vi "MH_WRabbitSetSFPData.vi"(6 "alphas":i32[](array[numeric]), 7 "sfpnames":string[](array[string]), 8 "error in (no error)":errorcluster, 9 "dRxs":i32[](array[numeric]), 10 "dTxs":i32[](array[numeric]), 11 "devidx":i32) -> (0 "error out":errorcluster, 3 "return type":i32)   [LabVIEW 2019]
uses:
  MH_DllPath_global.vi
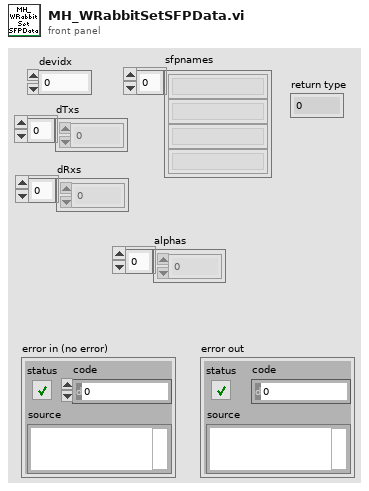
[diagram p1: front panel]
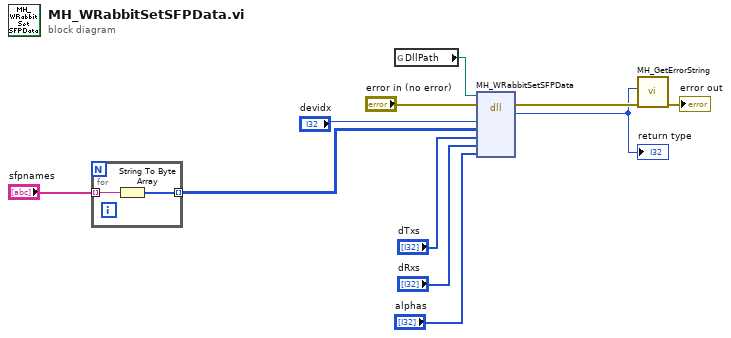
[diagram p0: block diagram]
diagram:
  n1 = for {
    tunnel: "sfpnames" -> [w13] mode=indexing
    tunnel: [w12] -> w1 mode=indexing
    n2 = String To Byte Array(string=w13) -> (unsigned byte array=w12:u8[])
  }
  n3 = global read "MH_DllPath_global.vi" "DllPath"() -> (w9:path)
  n4 = dll-call lib="MHLib64.dll" fn="MH_WRabbitSetSFPData"(path in=w9, error in="error in (no error)", "devidx"="devidx", "sfpnames"=w1, "dTxs"="dTxs", "dRxs"="dRxs", "alphas"="alphas") -> (error out=w8:errorcluster, "return type"=w7:i32)  [unwired: 6 in, 1 out]
  "return type" <- w7
  n5 = call "MH_GetErrorString.vi"("error in (no error)"=w8, "code"=w7) -> ("error out"=→"error out":errorcluster)  [unwired: 7 in, 2 out]
